vi "DefDataSave.vi"(0 "VISA IN":refnum<visa-resource-name>, 5 "error in":errorcluster) -> (14 "VISA Out":refnum<visa-resource-name>, 19 "error out":errorcluster)   [LabVIEW 2018, in "PNA-X.lvlib"]
uses:
  PNA-X.lvlib
panel:
  in  "Dsply":string(combo)="AUTO"
  in  "Traces":string(combo)="AUTO"
  in  "Format":string(combo)="AUTO"
  in  "FileType":string(combo)="CSA"
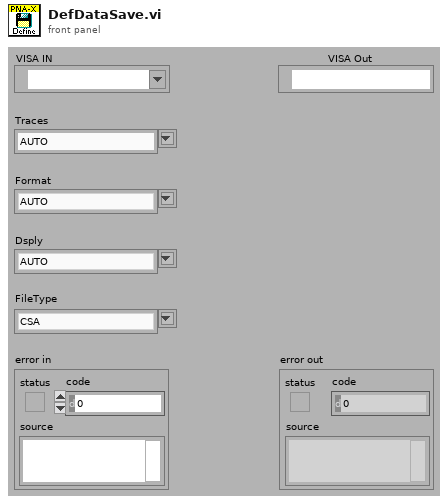
[diagram p1: front panel]
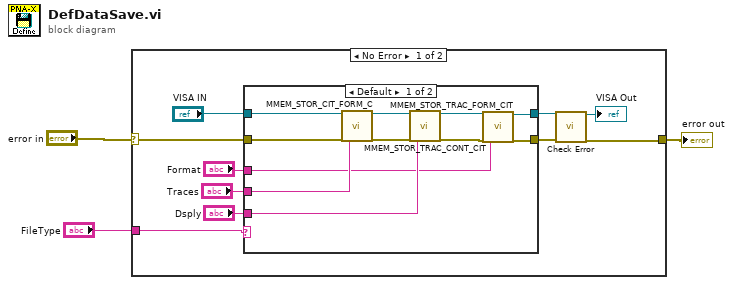
[diagram p0: block diagram]
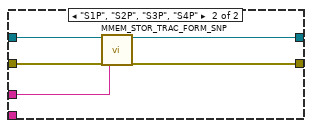
[diagram p2: hidden frame]
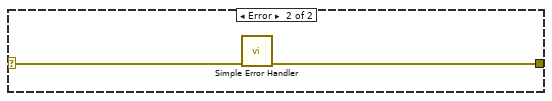
[diagram p3: hidden frame]
diagram:
  n1 = case shown="No Error" "error in" {
    selector: "error in" -> [w10 w31]
    tunnel: [w13 w30] -> w3
    tunnel: "FileType" -> [w11 _]
    frame No Error {
      n2 = case shown="Default" w11 {
        tunnel: w10 -> [w24 w29]
        tunnel: "VISA IN" -> [w23 w28]
        tunnel: [w15 w27] -> w7
        tunnel: [w14 w26] -> w8
        tunnel: "Format" -> [w16 w25]
        tunnel: "Traces" -> [w22 _]
        tunnel: "Dsply" -> [w20 _]
        frame Default {
          n3 = call "MMEM_STOR_CIT_FORM_C.vi"("VISA IN"=w23, "error in"=w24, "Traces"=w22) -> ("VISA Out"=w19:refnum<visa-resource-name>, "error out"=w21:errorcluster)  [unwired: 15 in]
          n4 = call "MMEM_STOR_TRAC_CONT_CIT.vi"("VISA IN"=w19, "error in"=w21, "Format"=w20) -> ("VISA Out"=w17:refnum<visa-resource-name>, "error out"=w18:errorcluster)  [unwired: 15 in]
          n5 = call "MMEM_STOR_TRAC_FORM_CIT.vi"("VISA IN"=w17, "error in"=w18, "Format"=w16) -> ("VISA Out"=w14:refnum<visa-resource-name>, "error out"=w15:errorcluster)  [unwired: 15 in]
        }
        frame "S1P", "S2P", "S3P", "S4P" {
          n6 = call "MMEM_STOR_TRAC_FORM_SNP.vi"("VISA IN"=w28, "error in"=w29, "Format"=w25) -> ("VISA Out"=w26:refnum<visa-resource-name>, "error out"=w27:errorcluster)  [unwired: 15 in]
        }
      }
      n7 = call "Check Error.vi"("VISA Resource Name"=w8, "error in (no error)"=w7) -> ("dup VISA session"=→"VISA Out":refnum<visa-resource-name>, "error out"=w13:errorcluster)  [unwired: 16 in]
    }
    frame Error {
      n8 = call <vilib>:"Simple Error Handler.vi"("error in (no error)"=w31) -> ("error out"=w30:errorcluster)  [unwired: 4 in, 4 out]
    }
  }
  "error out" <- w3
